vi "Ethernet Read.vi"(6 "connection ID":refnum<k5>, 7 "Stop Notification":refnum<notifier>, 8 "error in":errorcluster, 9 "Client Info":T1, 10 "TCP Engine Response Q":refnum<queue>, 11 "Main Engine Response Q":refnum<queue>) -> (0 "error out":errorcluster)   [LabVIEW 2024]
doc: "All Rights Reserved © 2017 SyncSols"
uses:
  Controls/Ethernet Client Info Cluster.ctl
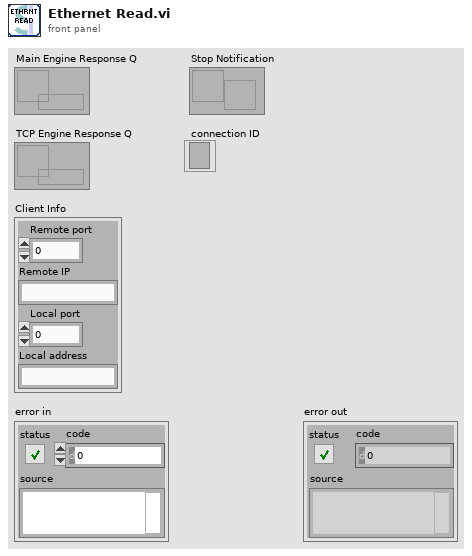
[diagram p1: front panel]
types:
  T1 = typedef "Ethernet Client Info Cluster.ctl" = cluster{"Remote port":u16, "Remote IP":string, "Local port":u16, "Local address":string}
  T2 = cluster{"Command":string, "SubCmd":string, "Data":cluster{"Remote IP":string, "Length":u16, "Data":u8[], "Remote port":u16, "Local IP":string, "Local port":u16, "Time":string}, "Protocol":string}
  T3 = cluster{"Command":string, "SubCmd":string, "Data":cluster{"Time":timestamp, "Client IP":string, "Length":u16, "Data":u8[], "Client Port":u16, "Server Port":u16, "Server IP":string}, "Protocol":string}
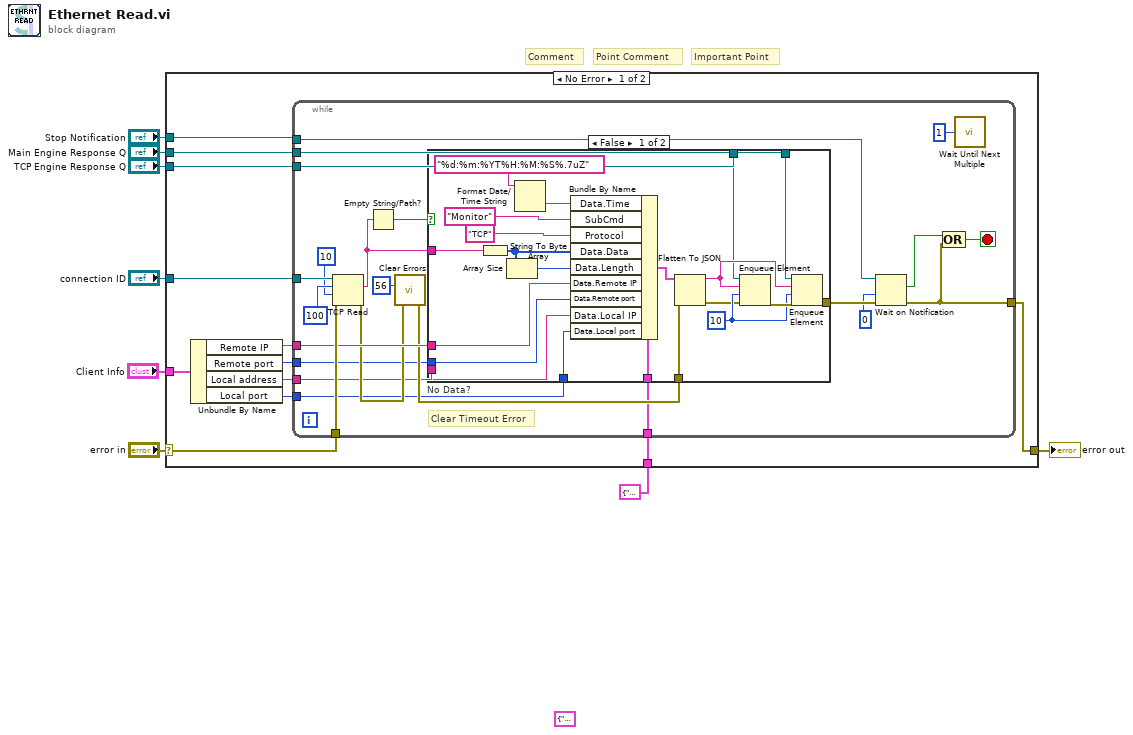
[diagram p0: block diagram]
diagram:
  (unwired) T3 {"Command"="", "SubCmd"="", "Data"={"Time"=timestamp(0 s since 1904-01-01), "Client IP"="", "Length"=0, "Data"=[], "Client Port"=0, "Server Port"=0, "Server IP"=""}, "Protocol"=""}
  # "Important Point"
  # "Point Comment"
  # "Comment"
  n1 = case shown="No Error" "error in" {
    selector: "error in" -> [w20 w66]
    tunnel: [w19 w66] -> w8
    tunnel: "Stop Notification" -> [w18 _]
    tunnel: "Main Engine Response Q" -> [w17 _]
    tunnel: "TCP Engine Response Q" -> [w16 _]
    tunnel: "Client Info" -> [w15 _]
    tunnel: "connection ID" -> [w12 _]
    tunnel: T2 {"Command"="Ethernet", "SubCmd"="", "Data"={"Remote IP"="", "Length"=0, "Data"=[], "Remote port"=0, "Local IP"="", "Local port"=0, "Time"=""}, "Protocol"=""} -> [w9 _]
    frame No Error {
      n2 = Unbundle By Name(w15) -> ("Remote IP"=w14:string, "Remote port"=w13:u16, "Local address"=w11:string, "Local port"=w10:u16)
      n3 = while {
        tunnel: w20 -> [w43]
        tunnel: [w38] -> w19
        tunnel: w14 -> [w36]
        tunnel: w17 -> [w35]
        tunnel: w16 -> [w34]
        tunnel: w18 -> [w33]
        tunnel: w13 -> [w29]
        tunnel: w12 -> [w28]
        tunnel: w11 -> [w25]
        tunnel: w10 -> [w24]
        tunnel: w9 -> [w21]
        stop <- w39 stop-if-true
        # "Clear Timeout Error"
        n4 = TCP Read(connection ID=w28, bytes to read=100 ("timeout ms (25000)"), error in (no error)=w43, 9:10 ("timeout ms (25000)")) -> (data out=w23:string, error out=w31:errorcluster)  [unwired: 1 in, 1 out]
        n5 = Empty String/Path?(string/path=w23) -> (empty?=w22:bool)
        n6 = call <vilib>:"Clear Errors.vi"("error in (no error)"=w31, "specific error code to clear (0: all)"=56) -> ("error out"=w30:errorcluster)  [unwired: 4 in, 1 out]
        n7 = case "No Data?" shown="False" w22 {
          tunnel: [w64 w65] -> w42
          tunnel: w36 -> [w54 _]
          tunnel: w35 -> [w53 _]
          tunnel: w34 -> [w52 _]
          tunnel: w30 -> [w51 w65]
          tunnel: w29 -> [w50 _]
          tunnel: w25 -> [w49 _]
          tunnel: w24 -> [w48 _]
          tunnel: w23 -> [w47 _]
          tunnel: w21 -> [w46 _]
          frame False {
            w62 = 10 ("timeout in ms (-1)")
            n8 = String To Byte Array(string=w47) -> (unsigned byte array=w56:u8[])
            n9 = Array Size(array=w56) -> (size(s)=w55:i32)
            n10 = Format Date/Time String(time format string (%c)="%d:%m:%YT%H:%M:%S%.7uZ") -> (date/time string=w44:string)  [unwired: 2 in]
            n11 = Bundle By Name(cluster=w46, "Data.Time"=w44, "SubCmd"="Monitor" ("Sub Command"), "Protocol"="TCP" ("Command"), "Data.Data"=w56, "Data.Length"=w55, "Data.Remote IP"=w54, "Data.Remote port"=w50, "Data.Local IP"=w49, "Data.Local port"=w48) -> (w59:T2)
            n12 = Flatten To JSON(anything=w59, error in (no error)=w51) -> (JSON string=w61:string, 11:w60:errorcluster)  [unwired: 1 in]
            n13 = Enqueue Element(queue=w52, element=w61, timeout in ms (-1)=w62, error in (no error)=w60) -> (error out=w63:errorcluster)  [unwired: 2 out]
            n14 = Enqueue Element(queue=w53, element=w61, timeout in ms (-1)=w62, error in (no error)=w63) -> (error out=w64:errorcluster)  [unwired: 2 out]
          }
          frame True {
          }
        }
        n15 = Wait on Notification(notifier=w33, timeout in ms (-1)=0, error in (no error)=w42) -> (notification=w40:bool, error out=w38:errorcluster)  [unwired: 1 in, 2 out]
        n16 = Compound Arithmetic op=OR(w40, w38) -> (w39:bool)
        n17 = call "Wait Until Next Multiple"("Count(mSec)"=u32 1) -> ()  [unwired: 1 out]
      }
    }
    frame Error {
    }
  }
  "error out" <- w8
